vi "MakeCommonPupilArray.vi"(8 "error in (no error)":errorcluster, 11 "HASO4_3 in":refnum<class "ILAO_BeamShaper.lvclass">) -> (0 "error out":errorcluster, 3 "HASO4_3 out":refnum<class "ILAO_BeamShaper.lvclass">)   [LabVIEW 2020]
uses:
  ILAO_BeamShaper.lvclass
  C:/GEECS/Developers Version/source/Device Drivers/BaseDriver/BaseDriver.lvclass
  C:/GEECS/Developers Version/source/Device Drivers/ILAO_BeamShaper/ILAO_BeamShaper/ILAO_BeamShaper.lvclass
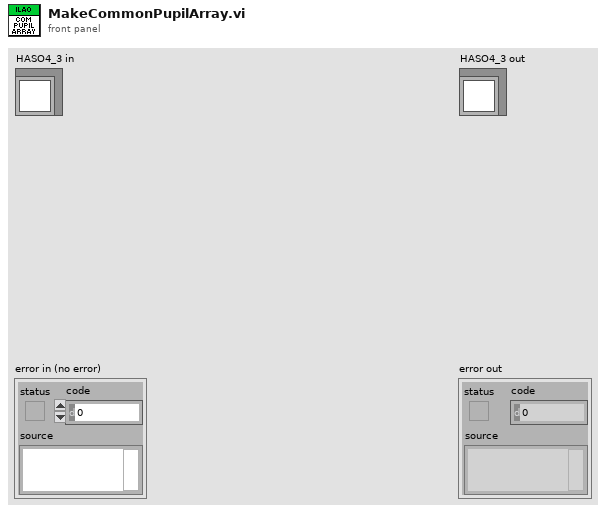
[diagram p1: front panel]
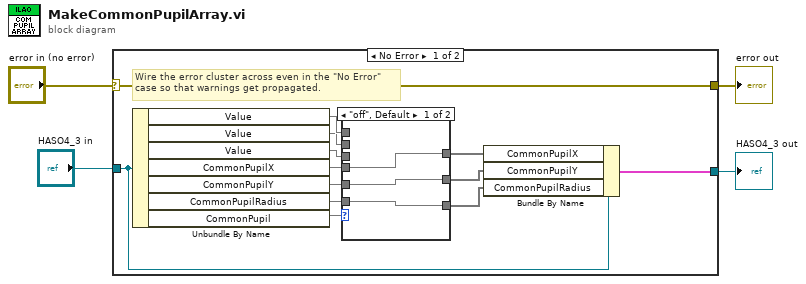
[diagram p0: block diagram]
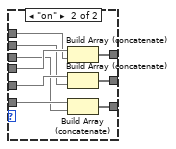
[diagram p2: hidden frame]
diagram:
  n1 = case shown="No Error" "error in (no error)" {
    selector: "error in (no error)" -> [w17 w31]
    tunnel: [w17 w31] -> w3
    tunnel: [w9 w30] -> w1
    tunnel: "HASO4_3 in" -> [w10 w30]
    frame No Error {
      # "Wire the error cluster across even in the \"No Error\"\ncase so that warnings get propagated."
      n2 = Unbundle By Name(w10) -> ("Value"=w15, "Value"=w13, "Value"=w11, "CommonPupilX"=w16, "CommonPupilY"=w14, "CommonPupilRadius"=w12, "CommonPupil"=w5)
      n3 = case shown="\"off\", Default" w5 {
        tunnel: w16 -> [w20 w29]
        tunnel: w15 -> [_ w28]
        tunnel: w14 -> [w19 w27]
        tunnel: w13 -> [_ w26]
        tunnel: w12 -> [w18 w25]
        tunnel: w11 -> [_ w24]
        tunnel: [w20 w23] -> w8
        tunnel: [w19 w22] -> w7
        tunnel: [w18 w21] -> w6
        frame "off", Default {
        }
        frame "on" {
          n4 = Build Array (concatenate)(w29, w28) -> (w23:void[])
          n5 = Build Array (concatenate)(w27, w26) -> (w22:void[])
          n6 = Build Array (concatenate)(w25, w24) -> (w21:void[])
        }
      }
      n7 = Bundle By Name(cluster=w10, "CommonPupilX"=w8, "CommonPupilY"=w7, "CommonPupilRadius"=w6) -> (w9:cluster{})
    }
    frame Error {
    }
  }
  "error out" <- w3
  "HASO4_3 out" <- w1
